vi "Run.vi"(8 "error in (no error)":errorcluster, 11 "angles in":refnum<class "angles.lvclass">) -> (0 "error out":errorcluster, 3 "angles out":refnum<class "angles.lvclass">)   [LabVIEW 2018, in "angles.lvclass"]
uses:
  angles.lvclass
  angles.lvclass/angles.ctl
  Device.lvclass
  StateMachine/State Machine.lvclass
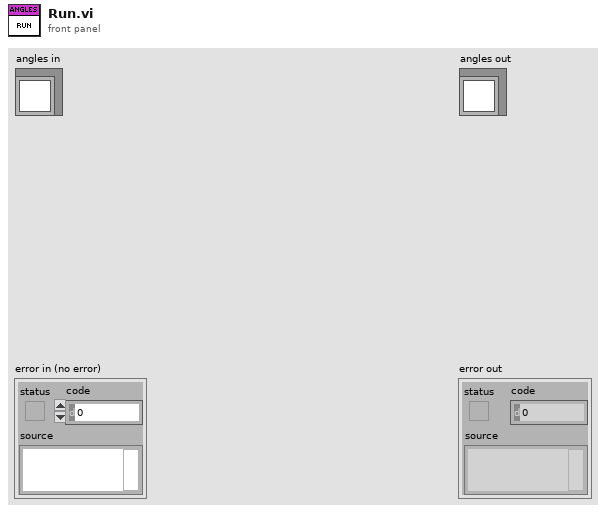
[diagram p1: front panel]
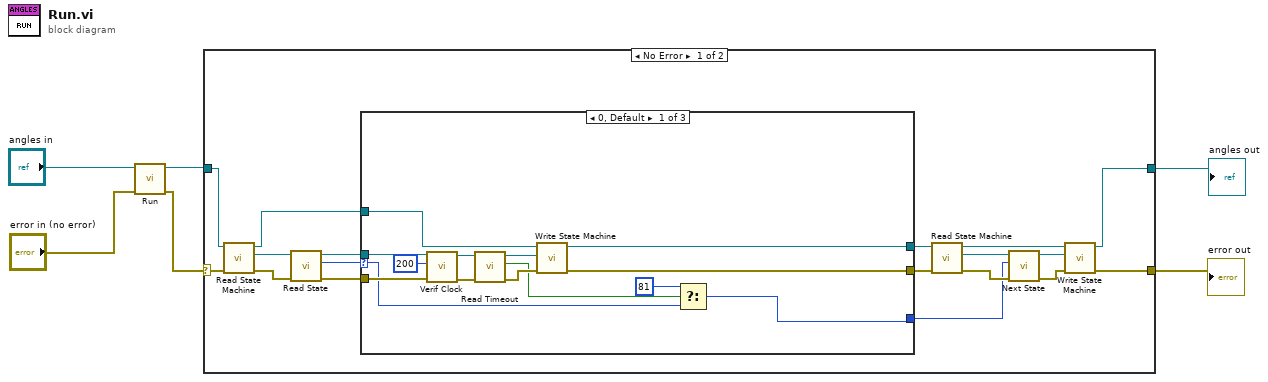
[diagram p0: block diagram]
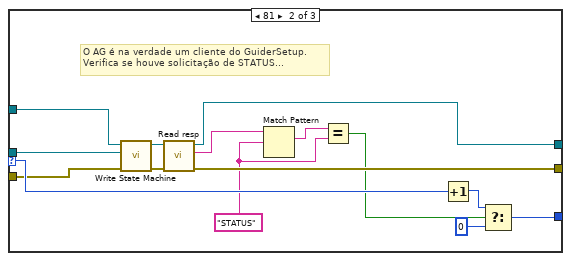
[diagram p2: hidden frame]
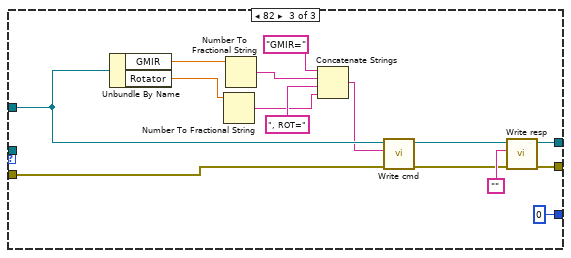
[diagram p3: hidden frame]
diagram:
  n1 = call-parent "Run.vi"("error in (no error)"="error in (no error)", "Device in"="angles in") -> ("error out"=w4:errorcluster, "Device out"=w3:refnum<class "angles.lvclass">)  [unwired: 8 in]
  n2 = case shown="No Error" w4 {
    selector: w4 -> [w23 w70]
    tunnel: [w15 w70] -> w1
    tunnel: w3 -> [w24 w69]
    tunnel: [w14 w69] -> w2
    frame No Error {
      n3 = call-dynamic "Read State Machine.vi"("error in (no error)"=w23, "Device in"=w24) -> ("error out"=w21:errorcluster, "State Machine.lvclass"=w22:refnum<class "State Machine.lvclass">, "Device out"=w12:refnum<class "angles.lvclass">)  [unwired: 7 in]
      n4 = call-dynamic "Read State.vi"("error in (no error)"=w21, "State Machine in"=w22) -> ("error out"=w11:errorcluster, "State"=w13:i32, "State Machine out"=w7:refnum<class "State Machine.lvclass">)  [unwired: 7 in]
      n5 = case shown="0, Default" w13 {
        selector: w13 -> [w26 w48 _]
        tunnel: w12 -> [w38 w51 w67]
        tunnel: w11 -> [w31 w43 w68]
        tunnel: [w34 w52 w56] -> w10
        tunnel: [w35 w53 w58] -> w9
        tunnel: [w25 w39 0 ("f")] -> w8
        tunnel: w7 -> [w33 w44 _]
        frame 0, Default {
          n6 = call-dynamic "Verif Clock.vi"("error in (no error)"=w31, "period"=u32 200, "State Machine in"=w33) -> ("error out"=w30:errorcluster, "State Machine out"=w32:refnum<class "State Machine.lvclass">)  [unwired: 7 in]
          n7 = call-dynamic "Read Timeout.vi"("error in (no error)"=w30, "State Machine in"=w32) -> ("error out"=w36:errorcluster, "Timeout"=w28:bool, "State Machine out"=w37:refnum<class "State Machine.lvclass">)  [unwired: 7 in]
          n8 = call-dynamic "Write State Machine.vi"("error in (no error)"=w36, "State Machine.lvclass"=w37, "Device in"=w38) -> ("error out"=w34:errorcluster, "Device out"=w35:refnum<class "angles.lvclass">)  [unwired: 7 in]
          n9 = Select(t=81 ("State"), s=w28, f=w26) -> (s? t:f=w25:i32)
        }
        frame 81 {
          w46 = "STATUS" ("regular expression")
          # "O AG é na verdade um cliente do GuiderSetup.\nVerifica se houve solicitação de STATUS..."
          n10 = call-dynamic "Write State Machine.vi"("error in (no error)"=w43, "State Machine.lvclass"=w44, "Device in"=w51) -> ("error out"=w49:errorcluster, "Device out"=w50:refnum<class "angles.lvclass">)  [unwired: 7 in]
          n11 = call-dynamic "Read resp.vi"("error in (no error)"=w49, "Device in"=w50) -> ("error out"=w52:errorcluster, "resp"=w45:string, "Device out"=w53:refnum<class "angles.lvclass">)  [unwired: 7 in]
          n12 = Match Pattern(string=w45, regular expression=w46) -> (match substring=w47:string)  [unwired: 1 in, 3 out]
          n13 = Equal?(x=w47, y=w46) -> (x = y?=w42:bool)
          n14 = Increment(x=w48) -> (x+1=w41:i32)
          n15 = Select(t=w41, s=w42, f=0) -> (s? t:f=w39:i32)
        }
        frame 82 {
          n16 = Unbundle By Name(w67) -> ("GMIR"=w66:dbl, "Rotator"=w65:dbl)
          n17 = Number To Fractional String(number=w65) -> (F-format string=w61:string)  [unwired: 3 in]
          n18 = Number To Fractional String(number=w66) -> (F-format string=w63:string)  [unwired: 3 in]
          n19 = Concatenate Strings("GMIR=" ("string"), w63, ", ROT=" ("string"), w61) -> (w60:string)
          n20 = call-dynamic "Write cmd.vi"("error in (no error)"=w68, "cmd"=w60, "Device in"=w67) -> ("error out"=w54:errorcluster, "Device out"=w55:refnum<class "angles.lvclass">)  [unwired: 7 in]
          n21 = call-dynamic "Write resp.vi"("error in (no error)"=w54, "resp"="", "Device in"=w55) -> ("error out"=w56:errorcluster, "Device out"=w58:refnum<class "angles.lvclass">)  [unwired: 7 in]
        }
      }
      n22 = call-dynamic "Read State Machine.vi"("error in (no error)"=w10, "Device in"=w9) -> ("error out"=w17:errorcluster, "State Machine.lvclass"=w19:refnum<class "State Machine.lvclass">, "Device out"=w18:refnum<class "angles.lvclass">)  [unwired: 7 in]
      n23 = call "Next State.vi"("error in (no error)"=w17, "New_State"=w8, "State Machine in"=w19) -> ("error out"=w16:errorcluster, "State Machine out"=w20:refnum<class "State Machine.lvclass">)  [unwired: 7 in]
      n24 = call-dynamic "Write State Machine.vi"("error in (no error)"=w16, "State Machine.lvclass"=w20, "Device in"=w18) -> ("error out"=w15:errorcluster, "Device out"=w14:refnum<class "angles.lvclass">)  [unwired: 7 in]
    }
    frame Error {
    }
  }
  "error out" <- w1
  "angles out" <- w2
